vi "Put Segment.vi"(8 "error in (no error)":errorcluster, 9 "Offset (-1)":i32=-1, 10 "Data":refnum<class "Array.lvclass">, 11 "TreeNode in":refnum<class "TreeNode.lvclass">) -> (0 "error out":errorcluster, 3 "TreeNode out":refnum<class "TreeNode.lvclass">)   [LabVIEW 2012, in "MDSplus.lvlib" / "TreeNode.lvclass"]
doc: "Write (part of) data segment."
uses:
  <vilib>/MDSplus/Classes/Data_Class/TreeNode_Class/TreeNode.lvclass
  <vilib>/MDSplus/Classes/Data_Class/Array_Class/Array.lvclass
  <vilib>/MDSplus/Classes/Data_Class/Data.lvclass
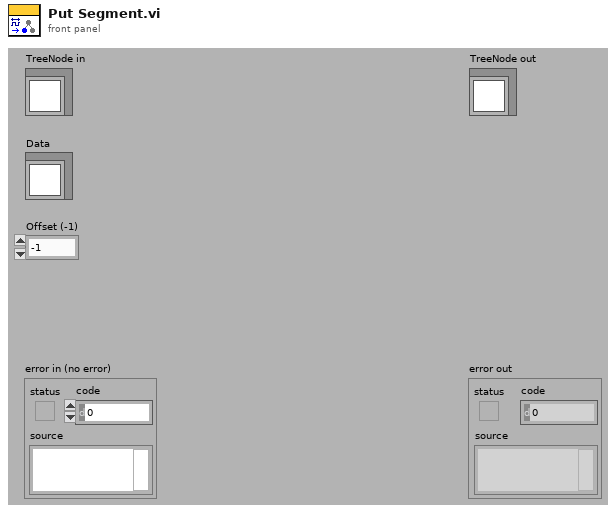
[diagram p1: front panel]
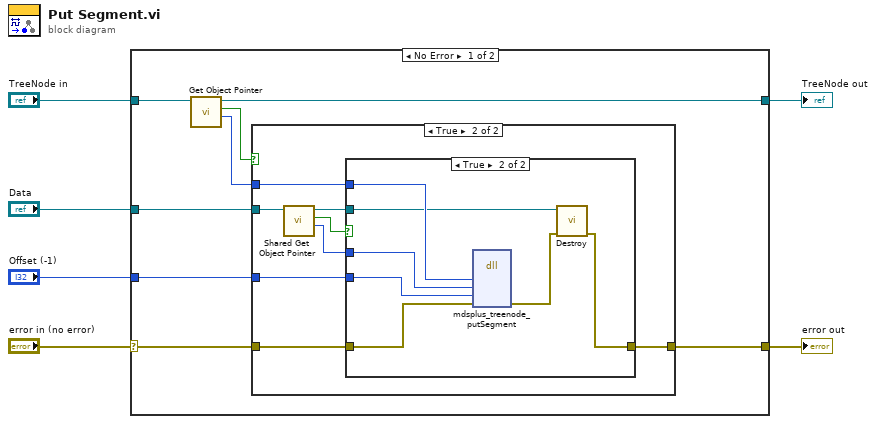
[diagram p0: block diagram]
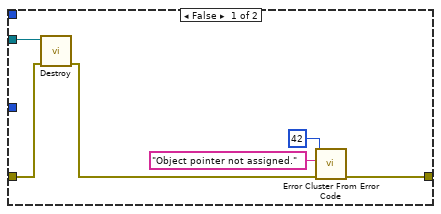
[diagram p2: hidden frame]
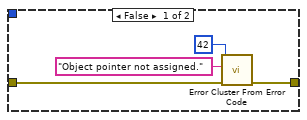
[diagram p3: hidden frame]
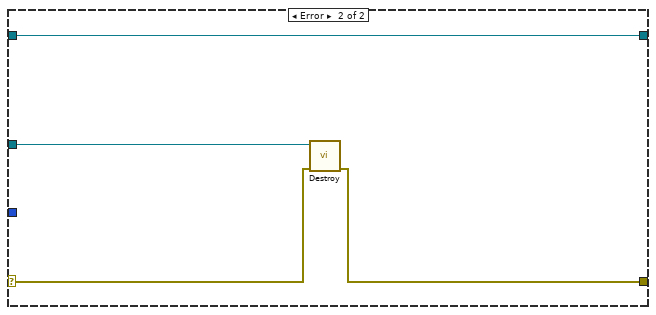
[diagram p4: hidden frame]
diagram:
  n1 = case shown="No Error" "error in (no error)" {
    selector: "error in (no error)" -> [w8 w41]
    tunnel: [w7 w40] -> w5
    tunnel: [w10 w43] -> w3
    tunnel: "TreeNode in" -> [w14 w43]
    tunnel: "Data" -> [w13 w42]
    tunnel: "Offset (-1)" -> [w9 _]
    frame No Error {
      n2 = call-dynamic "Get Object Pointer.vi"("Data in"=w14) -> ("Object Pointer"=w11:i64, "Assigned object pointer?"=w12:bool, "Data out"=w10:refnum<class "TreeNode.lvclass">)  [unwired: 8 in]
      n3 = case shown="True" w12 {
        tunnel: w13 -> [w18 w28]
        tunnel: w11 -> [_ w25]
        tunnel: w9 -> [_ w23]
        tunnel: w8 -> [w16 w22]
        tunnel: [w15 w21] -> w7
        frame False {
          n4 = call-dynamic "Destroy.vi"("error in (no error)"=w16, "Array in"=w18) -> ("error out"=w17:errorcluster)  [unwired: 9 in]
          n5 = call <vilib>:"Error Cluster From Error Code.vi"("error in (no error)"=w17, "error message (\"\")"="Object pointer not assigned." ("error message (\"\")"), "error code (0)"=42) -> ("error out"=w15:errorcluster)  [unwired: 6 in]
        }
        frame True {
          n6 = call <vilib>:"Shared Get Object Pointer.vi"("Data in"=w28) -> ("Object Pointer"=w26:i64, "Assigned object pointer?"=w27:bool, "Data out"=w24:refnum<class "Array.lvclass">)  [unwired: 8 in]
          n7 = case shown="True" w27 {
            tunnel: w26 -> [_ w38]
            tunnel: w25 -> [_ w39]
            tunnel: w24 -> [_ w37]
            tunnel: w23 -> [_ w35]
            tunnel: w22 -> [w30 w34]
            tunnel: [w29 w33] -> w21
            frame False {
              n8 = call <vilib>:"Error Cluster From Error Code.vi"("error in (no error)"=w30, "error message (\"\")"="Object pointer not assigned." ("error message (\"\")"), "error code (0)"=42) -> ("error out"=w29:errorcluster)  [unwired: 6 in]
            }
            frame True {
              n9 = dll-call lib="MDSobjectsLVShr" fn="mdsplus_treenode_putSegment"("lvTreeNodePtr"=w39, "lvDataPtrIn"=w38, "ofsIn"=w35, "error"=w34) -> ("error"=w36:errorcluster)  [unwired: 7 in, 2 out]
              n10 = call-dynamic "Destroy.vi"("error in (no error)"=w36, "Array in"=w37) -> ("error out"=w33:errorcluster)  [unwired: 9 in]
            }
          }
        }
      }
    }
    frame Error {
      n11 = call-dynamic "Destroy.vi"("error in (no error)"=w41, "Array in"=w42) -> ("error out"=w40:errorcluster)  [unwired: 9 in]
    }
  }
  "error out" <- w5
  "TreeNode out" <- w3
